vi "Enable Methods.vi"(10 "Method":string, 11 "LUnit Test Case In":refnum<class "LUnit Test Case.lvclass">) -> (3 "LUnit Test Case Out":refnum<class "LUnit Test Case.lvclass">)   [LabVIEW 2020, in "LUnit Test Case.lvclass"]
uses:
  LUnit Test Case.lvclass
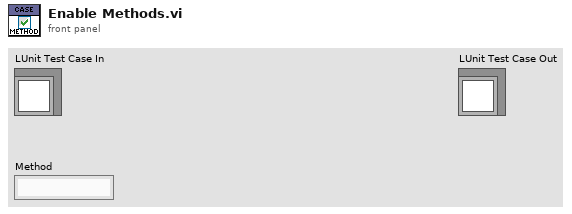
[diagram p1: front panel]
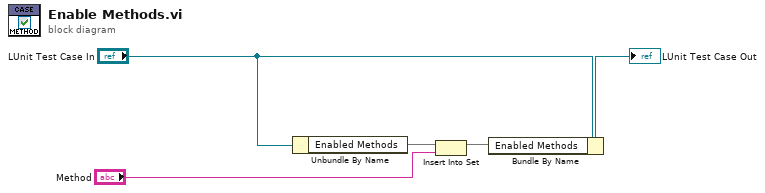
[diagram p0: block diagram]
diagram:
  n1 = Unbundle By Name("LUnit Test Case In") -> ("Enabled Methods"=w2:set{string})
  n2 = Insert Into Set(10:"Method", 11:w2) -> (3:w1:set{string})  [unwired: 1 out]
  n3 = Bundle By Name(cluster="LUnit Test Case In", "Enabled Methods"=w1) -> (→"LUnit Test Case Out":refnum<class "LUnit Test Case.lvclass">)
